vi "Scan_test.vi"(0 "DMM ref":refnum<visa-resource-name>, 1 "output cluster":cluster{"Timeout":i32, "Channel number":i32}, 2 "P_current_count":i32, 3 "N_current_count":i32, 5 "DMM error":errorcluster, 7 "Current Sense \nResitance Array":dbl[](array[numeric])=[1.0032214, 1.00250644, 1.00234822, 1.0040944, 1.0017711, 1.00229431, 1.00344206, 1.00482066, 1.00381056, 1.00290978, 1.00333016, 1.00367587], 9 "ESP32 ref":refnum<visa-resource-name>, 11 "ESP32 error":errorcluster, 12 "current_mode":u8[](array[numeric])=[0, 0, 0, 0, 0, 0, 0, 0, 0, 0, 0]) -> (4 "DMM ref":refnum<visa-resource-name>, 6 "DMM error":errorcluster, 8 "Measurements":dbl[](array[numeric]), 10 "ESP32 ref":refnum<visa-resource-name>, 13 "Timout?":bool, 14 "Time out count":i32, 15 "error out all":errorcluster[](array[cluster]))   [LabVIEW 2023]
uses:
  <instrlib>/Agilent 3446X Series/Agilent 3446X Series.lvlib
panel:
  out "ESP32 error":errorcluster
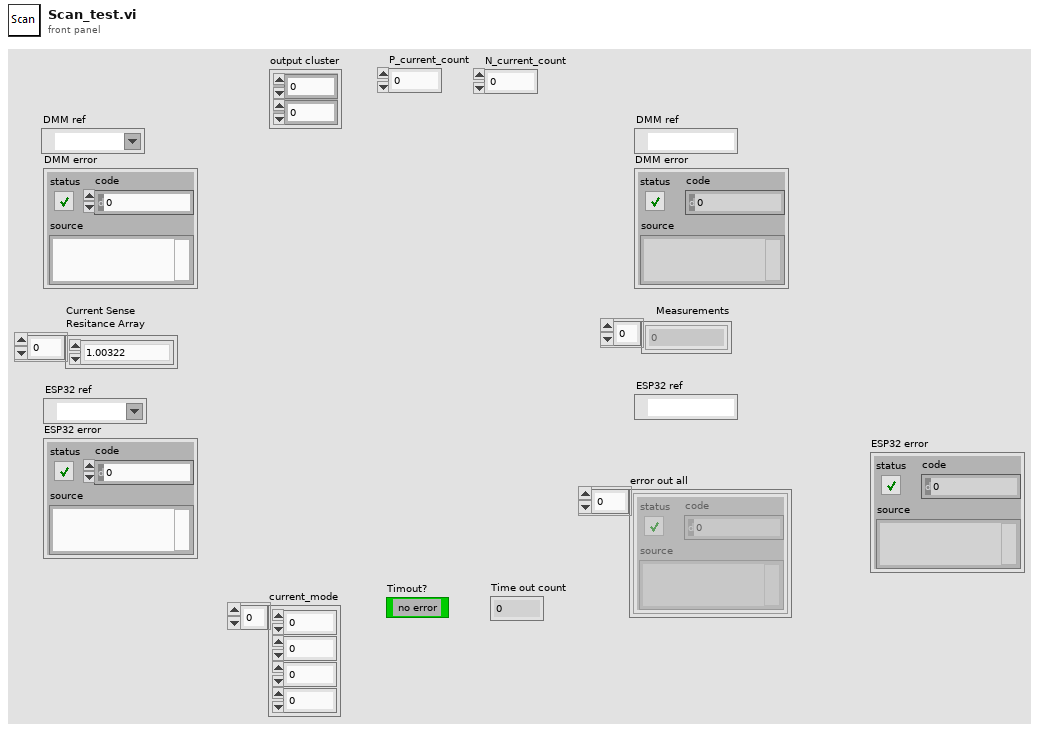
[diagram p1: front panel]
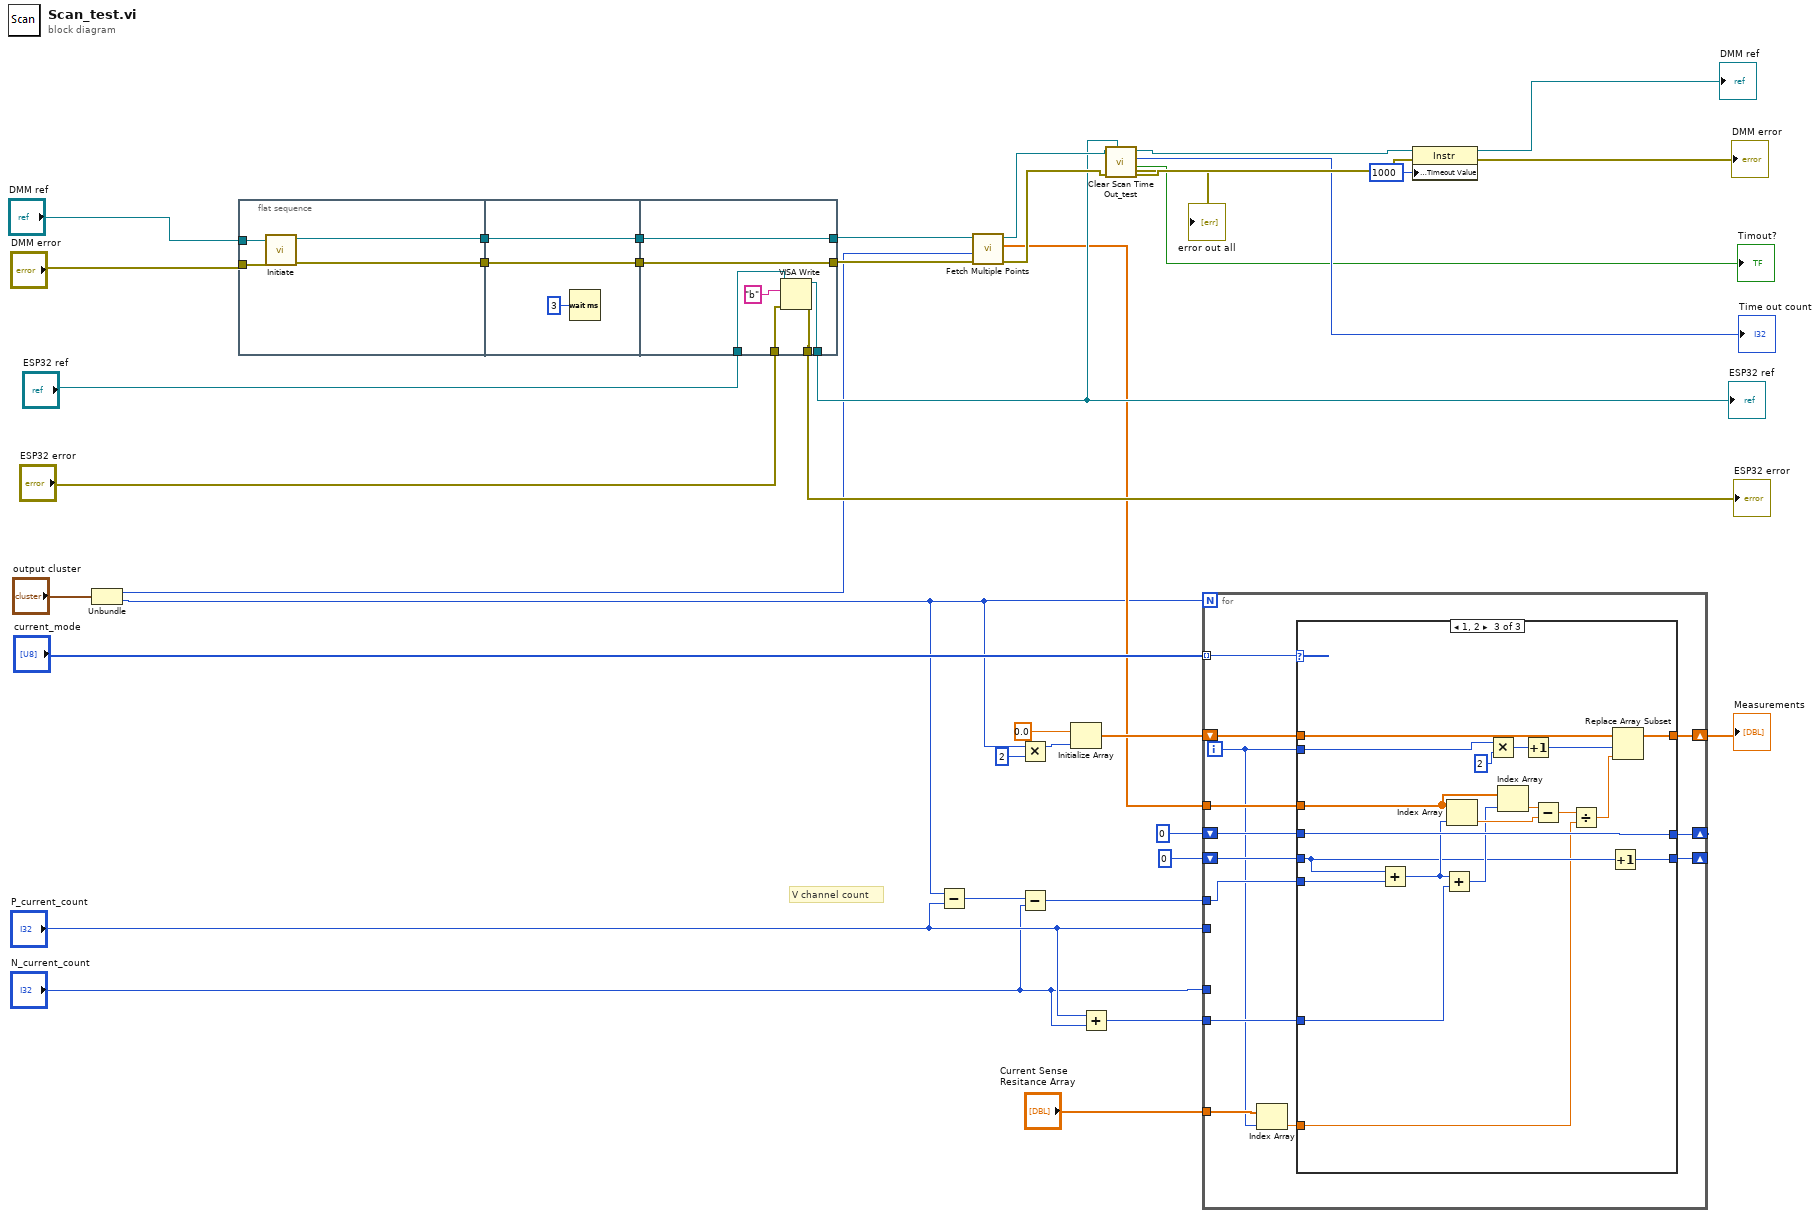
[diagram p0: block diagram]
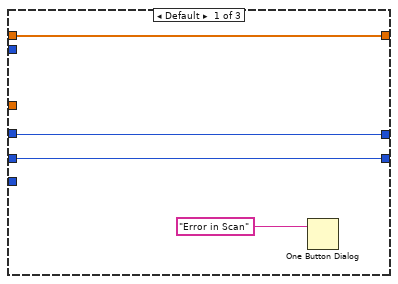
[diagram p2: hidden frame]
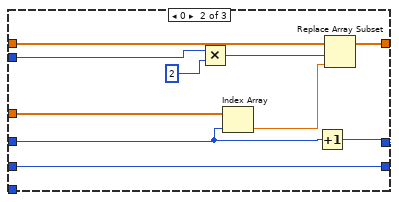
[diagram p3: hidden frame]
diagram:
  # "V channel count"
  n1 = Unbundle("output cluster") -> ("Timeout"=w2:i32, "Channel number"=w3:i32)
  n2 = flat-sequence {
    tunnel: [w44] -> w40
    tunnel: [w43] -> w39
    tunnel: "DMM ref" -> [w42]
    tunnel: "DMM error" -> [w41]
    tunnel: w40 -> [w47]
    tunnel: [w47] -> w38
    tunnel: w39 -> [w46]
    tunnel: [w46] -> w37
    tunnel: w38 -> [w54]
    tunnel: w37 -> [w53]
    tunnel: "ESP32 ref" -> [w52]
    tunnel: "ESP32 error" -> [w51]
    tunnel: [w50] -> w22
    tunnel: [w49] -> w23
    tunnel: [w54] -> w36
    tunnel: [w53] -> w35
    frame #0 {
      n3 = call <instrlib>:"Initiate.vi"("error in (no error)"=w41, "VISA resource name"=w42) -> ("error out"=w44:errorcluster, "VISA resource name out"=w43:refnum<visa-resource-name>)  [unwired: 8 in]
    }
    frame #1 {
      n4 = Wait (ms)(milliseconds to wait=u32 3) -> ()  [unwired: 1 out]
    }
    frame #2 {
      n5 = VISA Write(VISA resource name=w52, write buffer="b" ("data in"), error in (no error)=w51) -> (VISA resource name out=w50:refnum<visa-resource-name>, error out=w49:errorcluster)  [unwired: 1 out]
    }
  }
  n6 = Subtract(x=w3, y="P_current_count") -> (x-y=w13:i32)
  n7 = call <instrlib>:"Fetch Multiple Points.vi"("error in (no error)"=w36, "Timeout (10000 ms)"=w2, "VISA resource name"=w35) -> ("error out"=w31:errorcluster, "Measurements"=w14:dbl[], "VISA resource name out"=w32:refnum<visa-resource-name>)  [unwired: 1 in, 5 out]
  n8 = Multiply(x=w3, y=2) -> (x*y=w18:i32)
  n9 = Subtract(x=w13, y="N_current_count") -> (x-y=w12:i32)
  n10 = Initialize Array(0.0 ("Measurement"), w18) -> (w16:dbl[])
  n11 = Add(x="P_current_count", y="N_current_count") -> (x+y=w7:i32)
  n12 = call "Clear Scan Time Out_test.vi"("ESP32 ref"=w22, "error in (no error)"=w31, "VISA Refnum in"=w32) -> ("error out"=w29:errorcluster, "error?"=→"Timout?":bool, "Time out count"=→"Time out count":i32, "VISA Refnum out"=w30:refnum<visa-resource-name>, "error out all"=→"error out all":errorcluster[])  [unwired: 3 in, 1 out]
  n13 = for {
    N: w3 -> [_]
    shift-right: [w62] -> w6
    shift-left: w16 -> [w63]
    tunnel: "current_mode" -> [w67] mode=indexing
    tunnel: w14 -> [w66]
    tunnel: "P_current_count" -> [_]
    tunnel: "N_current_count" -> [_]
    tunnel: w12 -> [w59]
    shift-right: [w64] -> _
    shift-left: 0 ("index") -> [w65]
    shift-right: [w60] -> _
    shift-left: 0 ("index") -> [w61]
    tunnel: w7 -> [w58]
    tunnel: "Current Sense \nResitance Array" -> [w57]
    i -> [w56]
    n14 = Index Array(array=w57, index=w56) -> (element=w55:dbl)
    n15 = case shown="1, 2" w67 {
      tunnel: w66 -> [_ w81 w93]
      tunnel: w65 -> [w71 w79 w94]
      tunnel: [w71 w78 w94] -> w64
      tunnel: w56 -> [_ w76 w99]
      tunnel: w63 -> [w70 w77 w100]
      tunnel: [w70 w74 w96] -> w62
      tunnel: w61 -> [w69 w73 w86]
      tunnel: [w69 w73 w85] -> w60
      tunnel: w59 -> [_ _ w90]
      tunnel: w58 -> [_ _ w89]
      tunnel: w55 -> [_ _ w83]
      frame Default {
        n16 = One Button Dialog(message="Error in Scan") -> ()  [unwired: 1 in, 1 out]
      }
      frame 0 {
        n17 = Multiply(x=w76, y=2 ("x")) -> (x*y=w72:i32)
        n18 = Index Array(array=w81, index=w79) -> (element=w80:dbl)
        n19 = Increment(x=w79) -> (x+1=w78:i32)
        n20 = Replace Array Subset(array=w77, new element=w80, index=w72) -> (w74:dbl[])
      }
      frame 1, 2 {
        n21 = Add(x=w86, y=w90) -> (x+y=w88:i32)
        n22 = Add(x=w88, y=w89) -> (x+y=w87:i32)
        n23 = Index Array(array=w93, index=w88) -> (element=w91:dbl)
        n24 = Multiply(x=w99, y=2 ("x")) -> (x*y=w97:i32)
        n25 = Index Array(array=w93, index=w87) -> (element=w92:dbl)
        n26 = Increment(x=w97) -> (x+1=w95:i32)
        n27 = Subtract(x=w92, y=w91) -> (x-y=w84:dbl)
        n28 = Divide(x=w84, y=w83) -> (x/y=w82:dbl)
        n29 = Increment(x=w86) -> (x+1=w85:i32)
        n30 = Replace Array Subset(array=w100, new element=w82, index=w95) -> (w96:dbl[])
      }
    }
  }
  "Measurements" <- w6
  n31 = property class="Instr"(reference=w30, error in=w29, "General Settings:Timeout Value"=u32 1000) -> (reference out=→"DMM ref":refnum<visa-resource-name>, error out=→"DMM error":errorcluster)
  "ESP32 ref" <- w22
  "ESP32 error" <- w23
